vi "execution class name.vi"(8 "error in":errorcluster, 11 "fixed module parent implementation configuration in":refnum<class "control module configuration.lvclass">) -> (0 "error out":errorcluster, 2 "class name":string, 3 "fixed module parent implementation configuration out":refnum<class "control module configuration.lvclass">)   [LabVIEW 2013, in "control module configuration.lvclass"]
doc: "Provides an interface for determining the module runtime class associated with this module configuration. This class name can then be used to dynamically load or locate the runtime class for initialization purposes."
uses:
  control module configuration.lvclass
  <vilib>/NI/Tag Bus Module Framework/module configuration/TBM module configuration.lvclass
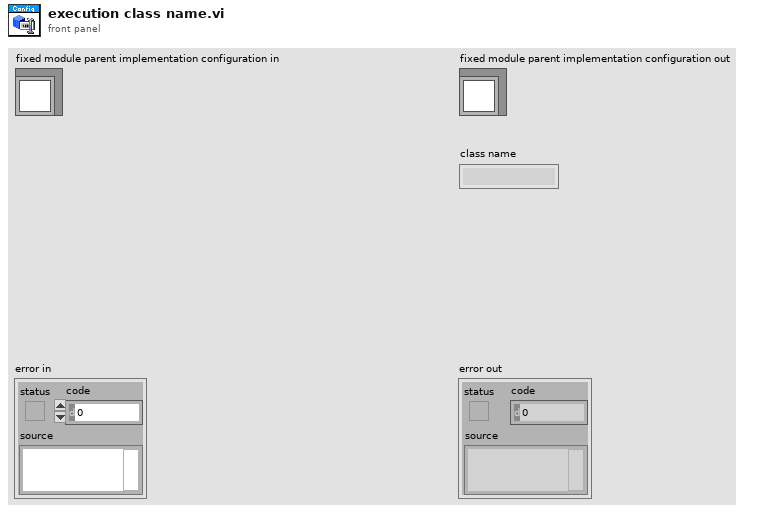
[diagram p1: front panel]
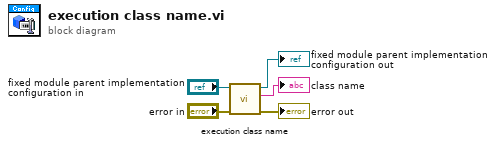
[diagram p0: block diagram]
diagram:
  n1 = call-parent "execution class name.vi"("error in"="error in", "configuration in"="fixed module parent implementation configuration in") -> ("error out"=→"error out":errorcluster, "execution class"=→"class name":string, "configuration out"=→"fixed module parent implementation configuration out":refnum<class "control module configuration.lvclass">)  [unwired: 7 in]
